vi "subtract average start.vi"(7 "data in":dbl[](array[numeric])) -> (8 "data with zero average out":dbl[](array[numeric]))   [LabVIEW 2019]
doc: "this subvi just subracts the average value of the data to make a data set with zero average."
uses:
  <vilib>/Analysis/baseanly.llb/Mean (DBL).vi
  <vilib>/Analysis/NI_AALBase.lvlib
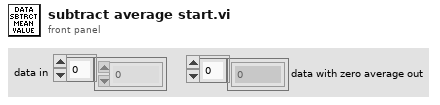
[diagram p1: front panel]
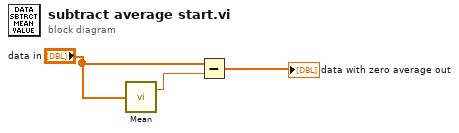
[diagram p0: block diagram]
diagram:
  n1 = call-poly <vilib>:"Mean.vi"("X"="data in") -> ("mean"=w2:dbl)  [unwired: 1 out]
  n2 = Subtract(x="data in", y=w2) -> (x-y=→"data with zero average out":dbl[])
